vi "InitAppearance.vi"(7 "Col Array Ref in":refnum<vi>, 8 "error in (no error)":errorcluster, 9 "Table Ref in":refnum<vi>, 10 "Col #":i32, 11 "MenuCol in":refnum<class "MenuCol.lvclass">) -> (0 "error out":errorcluster, 1 "Table Ref out":refnum<vi>, 3 "MenuCol out":refnum<class "MenuCol.lvclass">, 4 "Needs 2nd pass":bool)   [LabVIEW 2013, in "MenuCol.lvclass"]
doc: "Set column header, width, background and text color for entire table column."
uses:
  MenuCol.lvclass
  <vilib>/Utility/miscctls.llb/LVRowAndColumnTypeDef.ctl
  Column/Column.lvclass
  Column/Column.lvclass/Column.ctl
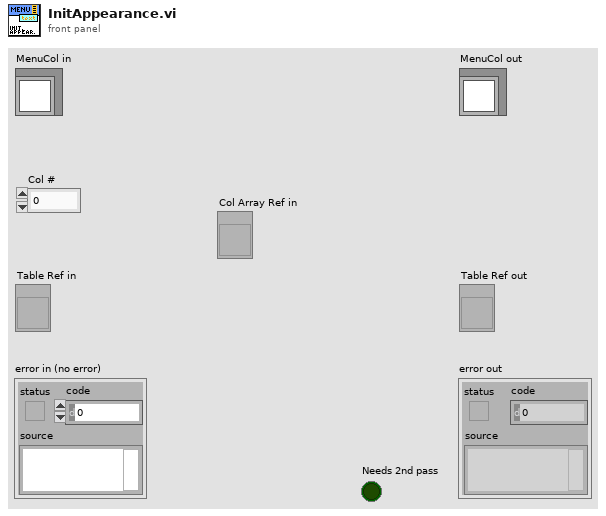
[diagram p1: front panel]
types:
  T1 = typedef "LVRowAndColumnTypeDef.ctl" = cluster{"Row":i32, "Column":i32}
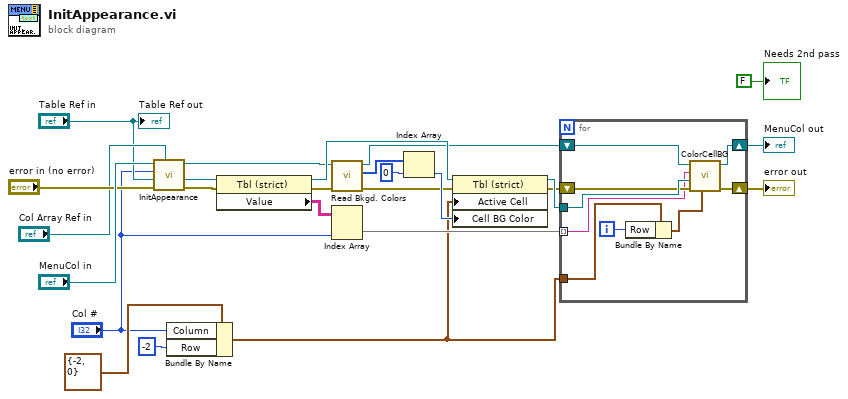
[diagram p0: block diagram]
diagram:
  n1 = call-parent "InitAppearance.vi"("Col Array Ref in"="Col Array Ref in", "error in (no error)"="error in (no error)", "Table Ref in"="Table Ref in", "Col #"="Col #", "Column in"="MenuCol in") -> ("error out"=w21:errorcluster, "Table Ref out"=w22:refnum<vi>, "Column out"=w5:refnum<class "MenuCol.lvclass">)  [unwired: 3 in, 1 out]
  n2 = Bundle By Name(cluster=T1 {"Row"=-2, "Column"=0} ("RowAndCollumn"), "Column"="Col #", "Row"=-2) -> (w2:T1)
  n3 = property class="Tbl (strict)"(reference=w22, error in=w21) -> (reference out=w13:refnum<vi>, error out=w6:errorcluster, "Value"=w24:string[][])
  n4 = call "Read Bkgd. Colors.vi"("error in (no error)"=w6, "Column in"=w5) -> ("error out"=w7:errorcluster, "Bkgd. Colors"=w10:u32[], "Column out"=w4:refnum<class "MenuCol.lvclass">)  [unwired: 7 in]
  n5 = Index Array(array=w24, index (col)="Col #") -> (element=w23:string[])  [unwired: 1 in]
  n6 = Index Array(array=w10, index=0) -> (element=w8:u32)
  n7 = property class="Tbl (strict)"(reference=w13, error in=w7, "Active Cell"=w2, "Cell BG Color"=w8) -> (reference out=w12:refnum<vi>, error out=w11:errorcluster)
  n8 = for {
    tunnel: w12 -> [w30]
    tunnel: w2 -> [w34]
    shift-right: [w28] -> w17
    shift-left: w11 -> [w29]
    tunnel: w23 -> [w26] mode=indexing
    shift-right: [w31] -> w16
    shift-left: w4 -> [w32]
    i -> [w33]
    n9 = Bundle By Name(cluster=w34, "Row"=w33) -> (w27:T1)
    n10 = call-dynamic "ColorCellBG.vi"("Cell Position"=w27, "error in (no error)"=w29, "Table CtlRef In"=w30, "Value"=w26, "MenuCol in"=w32) -> ("error out"=w28:errorcluster, "MenuCol out"=w31:refnum<class "MenuCol.lvclass">)  [unwired: 4 in, 1 out]
  }
  "error out" <- w17
  "MenuCol out" <- w16
  "Table Ref out" <- "Table Ref in"
  "Needs 2nd pass" <- FALSE ("Needs 2nd pass")
